vi "CMC_Dataflow.vi"() -> ()   [LabVIEW 2013]
doc: "A sample VI used to demonstrate dataflow."
panel:
  out "C 2":dbl
  in  "A 2":dbl=2.0
  out "C":dbl
  in  "B":dbl=3.0 min=0.0 max=100.0 step=1.0
  in  "A":dbl=2.0
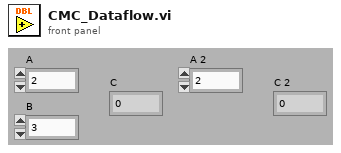
[diagram p1: front panel]
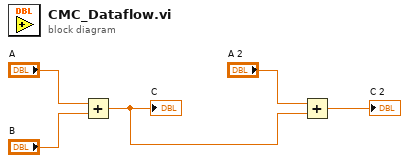
[diagram p0: block diagram]
diagram:
  n1 = Add(x="A", y="B") -> (x+y=w1:dbl)
  "C" <- w1
  n2 = Add(x="A 2", y=w1) -> (x+y=→"C 2":dbl)
